vi "Read Attributes.vi"(11 "Return File Path Msg":refnum<class "Return File Path Msg.lvclass">) -> (2 "Payload":cluster{"File Path":path})   [LabVIEW 2018, in "File Dialog Actor.lvlib" / "Return File Path Msg.lvclass"]
uses:
  Return File Path Msg.lvclass
  Return File Path Msg.lvclass/Return File Path Msg.ctl
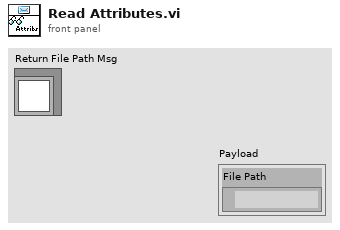
[diagram p1: front panel]
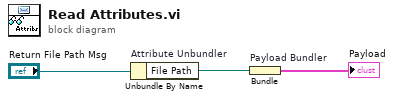
[diagram p0: block diagram]
diagram:
  n1 = Unbundle By Name "Attribute Unbundler"("Return File Path Msg") -> ("File Path"=w1:path)
  n2 = Bundle "Payload Bundler"("File Path"=w1) -> (→"Payload":cluster{"File Path":path})  [unwired: 1 in]
